vi "Victory Dialog.vi"(8 "error in (no error)":errorcluster, 10 "Victory Phrase":string) -> (0 "error out":errorcluster)   [LabVIEW 2014, in "SquareBattle.lvclass"]
uses:
  SquareBattle.lvclass
  Endigit Library/Endigit.lvlib
panel:
  in  "Finished":bool
  out "Victory Phrase out":string
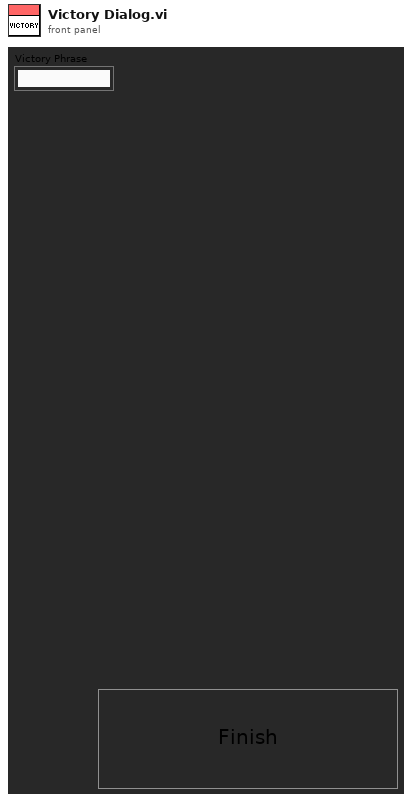
[diagram p1: front panel]
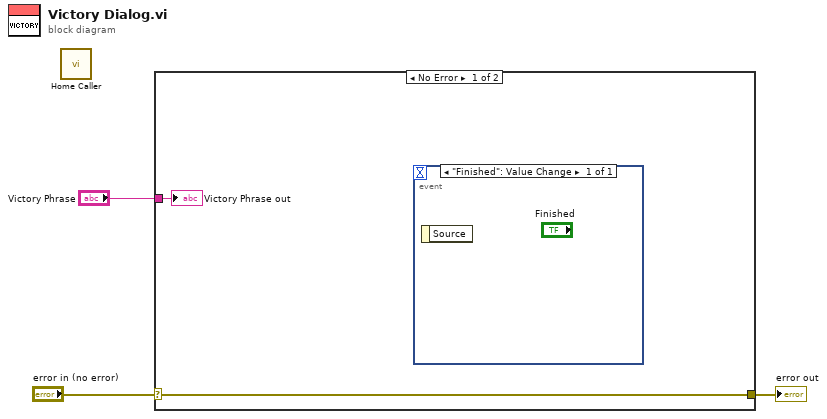
[diagram p0: block diagram]
diagram:
  n1 = call "Home Caller.vi"() -> ()  [unwired: 11 in]
  n2 = case shown="No Error" "error in (no error)" {
    selector: "error in (no error)" -> [w5 w6]
    tunnel: [w5 w6] -> w2
    tunnel: "Victory Phrase" -> [w4 _]
    frame No Error {
      n3 = event shown="[0] \"Finished\": Value Change" {
        selector: _ -> [_]
        dyn-events: _ -> [_]
        timeout: _ -> [_]
        event "Finished": Value Change {
          n4 = event-data() -> ()  [unwired: 1 in, 1 out]
        }
      }
      "Victory Phrase out" <- w4
    }
    frame Error {
    }
  }
  "error out" <- w2
